vi "Score and Rank Objects.vi"(6 "Targets":i32=3, 8 "Annotations":enum16{"None", "Good", "All"}(ring)=enum."Good", 9 "Score Limit":dbl=70.0, 10 "Object Info":T3(array[cluster]), 11 "Image in":T2) -> (0 "Object Info":T1(array[cluster]), 3 "Annotated Image":T2)   [LabVIEW 2020]
doc: "Use the location, size, and other factors to score and rank the objects. Optionally show annotations over the objects."
uses:
  <vilib>/vision/Image Controls.llb/IMAQ Image.ctl
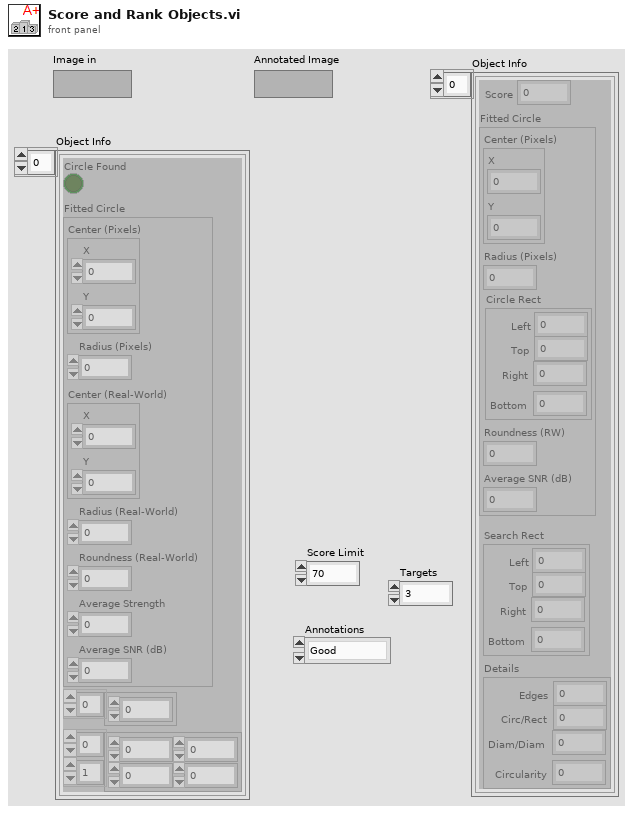
[diagram p1: front panel]
types:
  T1 = cluster{"Score":dbl, "Fitted Circle":cluster{"Center (Pixels)":cluster{"X":sgl, "Y":sgl}, "Radius (Pixels)":dbl, "Circle Rect":cluster{"Left":sgl, "Top":sgl, "Right":sgl, "Bottom":sgl}, "Roundness (RW)":dbl, "Average SNR (dB)":dbl}, "Search Rect":cluster{"Left":sgl, "Top":sgl, "Right":sgl, "Bottom":sgl}, "Details":cluster{"Edges":sgl, "Circ/Rect":sgl, "Diam/Diam":sgl, "Circularity":sgl}}[]
  T2 = typedef "IMAQ Image.ctl" = refnum<image>
  T3 = cluster{"Circle Found":bool, "Fitted Circle":cluster{"Center (Pixels)":cluster{"X":sgl, "Y":sgl}, "Radius (Pixels)":dbl, "Center (Real-World)":cluster{"X":sgl, "Y":sgl}, "Radius (Real-World)":dbl, "Roundness (Real-World)":dbl, "Average Strength":dbl, "Average SNR (dB)":dbl}, dbl[], dbl[][]}[]
  T4 = cluster{"Score":dbl, "Fitted Circle":cluster{"Center (Pixels)":cluster{"X":sgl, "Y":sgl}, "Radius (Pixels)":dbl, "Rect":cluster{"Left":sgl, "Top":sgl, "Right":sgl, "Bottom":sgl}, "Roundness (RW)":dbl, "Average SNR (dB)":dbl}, "Rect":cluster{"Left":sgl, "Top":sgl, "Right":sgl, "Bottom":sgl}, "Details":cluster{"Edges":sgl, "Circ/Rect":sgl, "Diam/Diam":sgl, "Circularity":sgl}}[]
  T5 = cluster{"Desired Font (Application)":enum16{"User-specified Font", "Application Font", "System Font", "Dialog Font"}, "[User-specified Font]":cluster{"Font Name":string, "Size":i16, "Strikeout?":bool, "Italic?":bool, "Underline?":bool, "Outline?":bool, "Shadow?":bool, "Bold?":bool, "Rotation Angle":dbl}, "Horizontal Alignment":i16, "Vertical Alignment":i16}
  T6 = cluster{"Center (Pixels)":cluster{"X":sgl, "Y":sgl}, "Radius (Pixels)":dbl, "Circle Rect":cluster{"Left":sgl, "Top":sgl, "Right":sgl, "Bottom":sgl}, "Roundness (RW)":dbl, "Average SNR (dB)":dbl}
  T7 = cluster{"Left":sgl, "Top":sgl, "Right":sgl, "Bottom":sgl}
  T8 = cluster{"Edges":sgl, "Circ/Rect":sgl, "Diam/Diam":sgl, "Circularity":sgl}
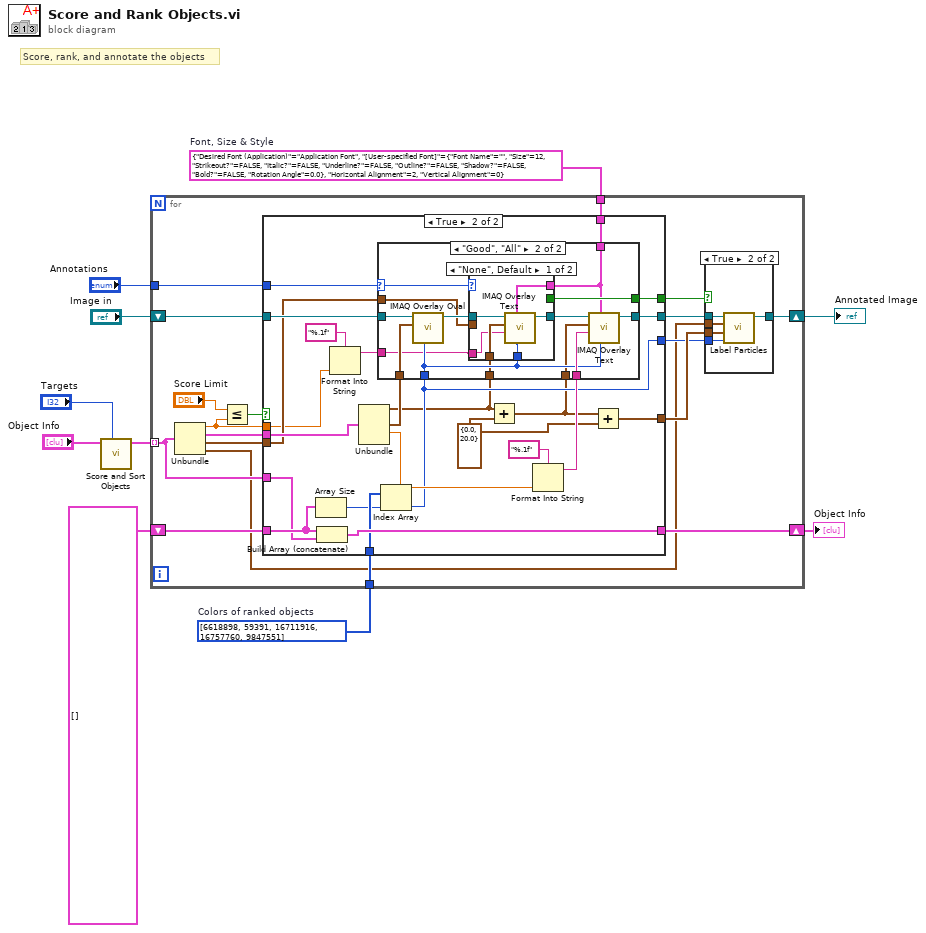
[diagram p0: block diagram]
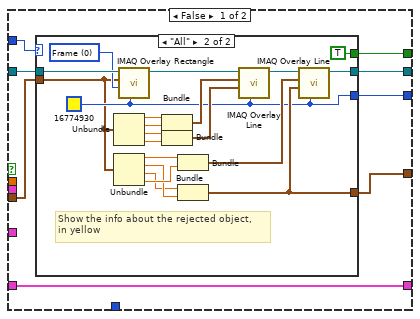
[diagram p3: hidden frame]
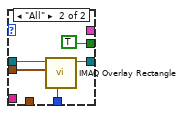
[diagram p6: hidden frame]
diagram:
  w8 = T5 {"Desired Font (Application)"=enum."Application Font", "[User-specified Font]"={"Font Name"="", "Size"=12, "Strikeout?"=FALSE, "Italic?"=FALSE, "Underline?"=FALSE, "Outline?"=FALSE, "Shadow?"=FALSE, "Bold?"=FALSE, "Rotation Angle"=0.0}, "Horizontal Alignment"=2, "Vertical Alignment"=0}  # Font, Size & Style
  w7 = u32[] [6618898, 59391, 16711916, 16757760, 9847551]  # Colors of ranked objects
  # "Score, rank, and annotate the objects"
  n1 = call "Score and Sort Objects.vi"("Targets"="Targets", "Object Info"="Object Info") -> ("Object Info"=w4:T1)  [unwired: 9 in]
  n2 = for {
    tunnel: w4 -> [w15] mode=indexing
    shift-right: [w26] -> w9
    shift-left: "Image in" -> [w25]
    shift-right: [w24] -> w3
    shift-left: T4 [] ("Object Info") -> [w23]
    tunnel: w8 -> [w22]
    tunnel: w7 -> [w21]
    tunnel: "Annotations" -> [w17]
    n3 = Unbundle(w15) -> ("Score"=w12:dbl, "Fitted Circle"=w27:T6, "Search Rect"=w28:T7, "Details"=w11:T8)
    n4 = Less Or Equal?(x="Score Limit", y=w12) -> (x <= y?=w13:bool)
    n5 = case shown="True" w13 {
      tunnel: w27 -> [_ w77]
      tunnel: w25 -> [w42 w87]
      tunnel: [w36 w86] -> w24
      tunnel: w28 -> [w41 w74]
      tunnel: [w40 w85] -> w20
      tunnel: w22 -> [_ w80]
      tunnel: w21 -> [_ w82]
      tunnel: [w39 w79] -> w19
      tunnel: w17 -> [w38 w72]
      tunnel: [w37 w73] -> w18
      tunnel: w23 -> [w36 w78]
      tunnel: [w35 w71] -> w16
      tunnel: w15 -> [_ w70]
      tunnel: w12 -> [_ w64]
      frame False {
        n6 = case shown="\"All\"" w38 {
          tunnel: w42 -> [w43 w63]
          tunnel: w41 -> [_ w45]
          tunnel: [w43 w48] -> w40
          tunnel: [_ w47] -> w39
          tunnel: [_ w46] -> w37
          tunnel: [_ TRUE] -> w35
          frame "None", Default {
            # "Rejected, not supposed to annotate"
          }
          frame "All" {
            w50 = u32 0 items=["Frame", "Fill", "Highlight"] ("Drawing Mode (Frame)")
            w46 = u32 16774930 ("Color")
            # "Show the info about the rejected object,\nin yellow"
            n7 = Unbundle(w45) -> ("Left"=w60:sgl, "Top"=w59:sgl, "Right"=w58:sgl, "Bottom"=w57:sgl)
            n8 = Unbundle(w45) -> ("Left"=w56:sgl, "Top"=w54:sgl, "Right"=w53:sgl, "Bottom"=w55:sgl)
            n9 = call "IMAQ Overlay Rectangle"("Color"=w46, "Drawing Mode (Frame)"=w50, "Rectangle"=w45, "Image"=w63) -> ("Image Out"=w62:T2)  [unwired: 6 in, 1 out]
            n10 = Bundle("Left"=w60, "Top"=w59) -> (w49:cluster{"Left":sgl, "Top":sgl})  [unwired: 1 in]
            n11 = Bundle("Right"=w58, "Bottom"=w57) -> (w52:cluster{"Right":sgl, "Bottom":sgl})  [unwired: 1 in]
            n12 = Bundle("Left"=w56, "Bottom"=w55) -> (w51:cluster{"Left":sgl, "Bottom":sgl})  [unwired: 1 in]
            n13 = Bundle("Right"=w53, "Top"=w54) -> (w47:cluster{"Right":sgl, "Top":sgl})  [unwired: 1 in]
            n14 = call "IMAQ Overlay Line"("Color"=w46, "End Point"=w52, "Start Point"=w49, "Image"=w62) -> ("Image Out"=w61:T2)  [unwired: 6 in, 1 out]
            n15 = call "IMAQ Overlay Line"("Color"=w46, "End Point"=w47, "Start Point"=w51, "Image"=w61) -> ("Image Out"=w48:T2)  [unwired: 6 in, 1 out]
          }
        }
      }
      frame True {
        w65 = cluster{dbl, dbl} {0.0, 20.0} ("x+y")
        n16 = Array Size(array=w78) -> (size(s)=w81:i32)
        n17 = Build Array (concatenate)(w78, w70) -> (w86:T1)
        n18 = Format Into String(format string="%.1f", w64) -> (resulting string=w68:string)  [unwired: 2 in, 1 out]
        n19 = Unbundle(w77) -> ("Center (Pixels)"=w66:cluster{"X":sgl, "Y":sgl}, "Circle Rect"=w76:T7, "Roundness (RW)"=w75:dbl)  [unwired: 2 out]
        n20 = Index Array(array=w82, index=w81) -> (element=w73:u32)
        n21 = Add(x=w66, y=w65) -> (x+y=w67:cluster{dbl, dbl})
        n22 = Format Into String(format string="%.1f", w75) -> (resulting string=w83:string)  [unwired: 2 in, 1 out]
        n23 = case shown="\"Good\", \"All\"" w72 {
          selector: w72 -> [_ w93]
          tunnel: w87 -> [w88 w102]
          tunnel: [w88 w100] -> w85
          tunnel: w83 -> [_ w99]
          tunnel: w80 -> [_ w91]
          tunnel: w73 -> [_ w97]
          tunnel: w67 -> [_ w96]
          tunnel: w76 -> [_ w95]
          tunnel: w74 -> [_ w94]
          tunnel: [_ w92] -> w71
          tunnel: w66 -> [_ w90]
          tunnel: w68 -> [_ w89]
          frame "None", Default {
          }
          frame "Good", "All" {
            n24 = call "IMAQ Overlay Oval"("Color"=w97, "Bounding Rectangle"=w95, "Image"=w102) -> ("Image Out"=w101:T2)  [unwired: 7 in, 1 out]
            n25 = case shown="\"None\", Default" w93 {
              tunnel: w94 -> [_ w113]
              tunnel: w101 -> [w108 w112]
              tunnel: [w107 w111] -> w98
              tunnel: w97 -> [w106 w110]
              tunnel: [_ TRUE] -> w92
              tunnel: w91 -> [w105 _]
              tunnel: w90 -> [w104 _]
              tunnel: w89 -> [w103 _]
              frame "None", Default {
                n26 = call "IMAQ Overlay Text"("Text Color (black)"=w106, "Font, Size & Style"=w105, "String"=w103, "Origin"=w104, "Image"=w108) -> ("Image Out"=w107:T2)  [unwired: 5 in, 1 out]
              }
              frame "All" {
                n27 = call "IMAQ Overlay Rectangle"("Color"=w110, "Rectangle"=w113, "Image"=w112) -> ("Image Out"=w111:T2)  [unwired: 7 in, 1 out]
              }
            }
            n28 = call "IMAQ Overlay Text"("Text Color (black)"=w97, "Font, Size & Style"=w91, "String"=w99, "Origin"=w96, "Image"=w98) -> ("Image Out"=w100:T2)  [unwired: 5 in, 1 out]
          }
        }
        n29 = Add(x=w67, y=w65) -> (x+y=w79:cluster{dbl, dbl})
      }
    }
    n30 = case shown="True" w16 {
      tunnel: [w29 w34] -> w26
      tunnel: w20 -> [w29 w33]
      tunnel: w19 -> [_ w32]
      tunnel: w18 -> [_ w31]
      tunnel: w11 -> [_ w30]
      frame False {
      }
      frame True {
        n31 = call "Label Particles.vi"("Color"=w31, "Location"=w32, "Details"=w30, "Image"=w33) -> ("Image 2"=w34:T2)  [unwired: 7 in]
      }
    }
  }
  "Annotated Image" <- w9
  "Object Info" <- w3
